vi "String Array to Comma Separated String.vi"(1 "String Array":string[](array[string])) -> (0 "comma separated string":string)   [LabVIEW 2020]
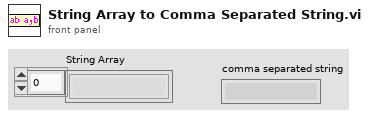
[diagram p1: front panel]
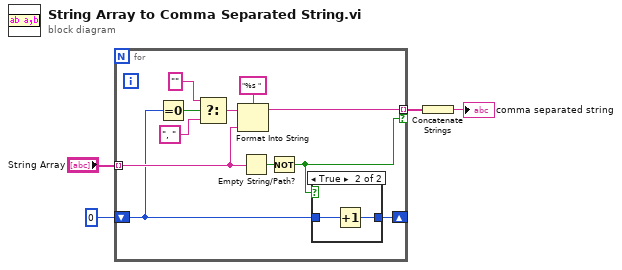
[diagram p0: block diagram]
diagram:
  n1 = for {
    tunnel: "String Array" -> [w9] mode=indexing
    tunnel: [w10] -> w3 mode=indexing if=w7
    shift-right: [w5] -> _
    shift-left: 0 -> [w6]
    n2 = Equal To 0?(x=w6) -> (x = 0?=w14:bool)
    n3 = Select(t="", s=w14, f=", ") -> (s? t:f=w11:string)
    n4 = Format Into String(format string="%s ", initial string=w11, w9) -> (resulting string=w10:string)  [unwired: 1 in, 1 out]
    n5 = Empty String/Path?(string/path=w9) -> (empty?=w8:bool)
    n6 = Not(x=w8) -> (.not. x?=w7:bool)
    n7 = case shown="True" w7 {
      tunnel: w6 -> [w16 w18]
      tunnel: [w16 w17] -> w5
      frame False {
      }
      frame True {
        n8 = Increment(x=w18) -> (x+1=w17:i32)
      }
    }
  }
  n9 = Concatenate Strings(w3) -> (→"comma separated string":string)
